vi "ATSh_SetCaptureClock.vi"(6 "Decimation":u32, 8 "Edge":u32, 9 "Rate":u32, 10 "Source":u32, 11 "Handle":u32) -> (0 "Return":u32, 3 "Handle_Out":u32)   [LabVIEW 2010]
doc: "_____AlazarTech, Scope_____\n\nConfigure the capture clock circuitry.\nHandle input.\n\nSource:\n - 0x1: INTERNAL\n - 0x2 : EXTERNAL\nRate: \n - 1KSPS 0x001\n - 2KSPS 0x002\n - 5KSPS 0x004\n - 10KSPS 0x008\n - 20KSPS 0x00A\n - 50KSPS 0x00C\n -100KSPS 0x00E\n -200KSPS 0x010\n -500KSPS 0x012\n - 1MSPS 0x014\n - 2MSPS 0x018\n - 5MSPS 0x01A\n - 10MSPS 0x01C\n - 20MSPS 0x01E\n - 25MSPS 0x021\n - 50MSPS 0x022\n -100MSPS 0x024\n -125MSPS 0x025\n -160MSPS 0x026\n -180MSPS 0x027\n -200MSPS 0x028\n -250MSPS 0x02B\n -500MSPS 0x030\n - 1GSPS 0x035\nEdge: \n - 0x0 : Rising\n - 0x1 : Falling \nDecimation: default 0"
uses:
  ATSApi.dll
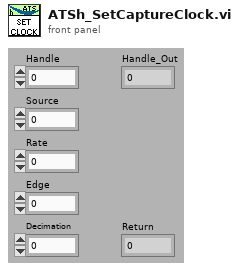
[diagram p1: front panel]
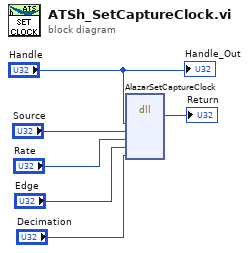
[diagram p0: block diagram]
diagram:
  n1 = dll-call lib="ATSApi.dll" fn="AlazarSetCaptureClock"("h"="Handle", "Source"="Source", "Rate"="Rate", "Edge"="Edge", "Decimation"="Decimation") -> (→"Return":u32)  [unwired: 8 in, 2 out]
  "Handle_Out" <- "Handle"
